vi "_033.vi"() -> ()   [LabVIEW 2024]
panel:
  out "Min":dbl
  out "Max":dbl
  in  "Array 4":dbl[](array[numeric])
  out "sum":dbl
  in  "Array 3":dbl[](array[numeric])
  out "x != 0?":bool
  out "x = 0?":bool
  in  "Numeric":dbl
  out "Array 2":dbl[](array[numeric])
  out "Array":dbl[](array[numeric])
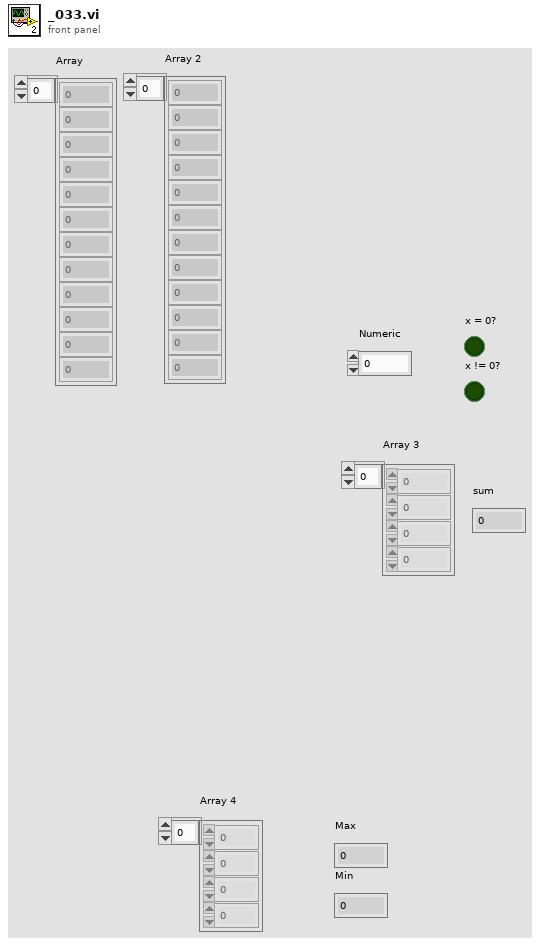
[diagram p1: front panel]
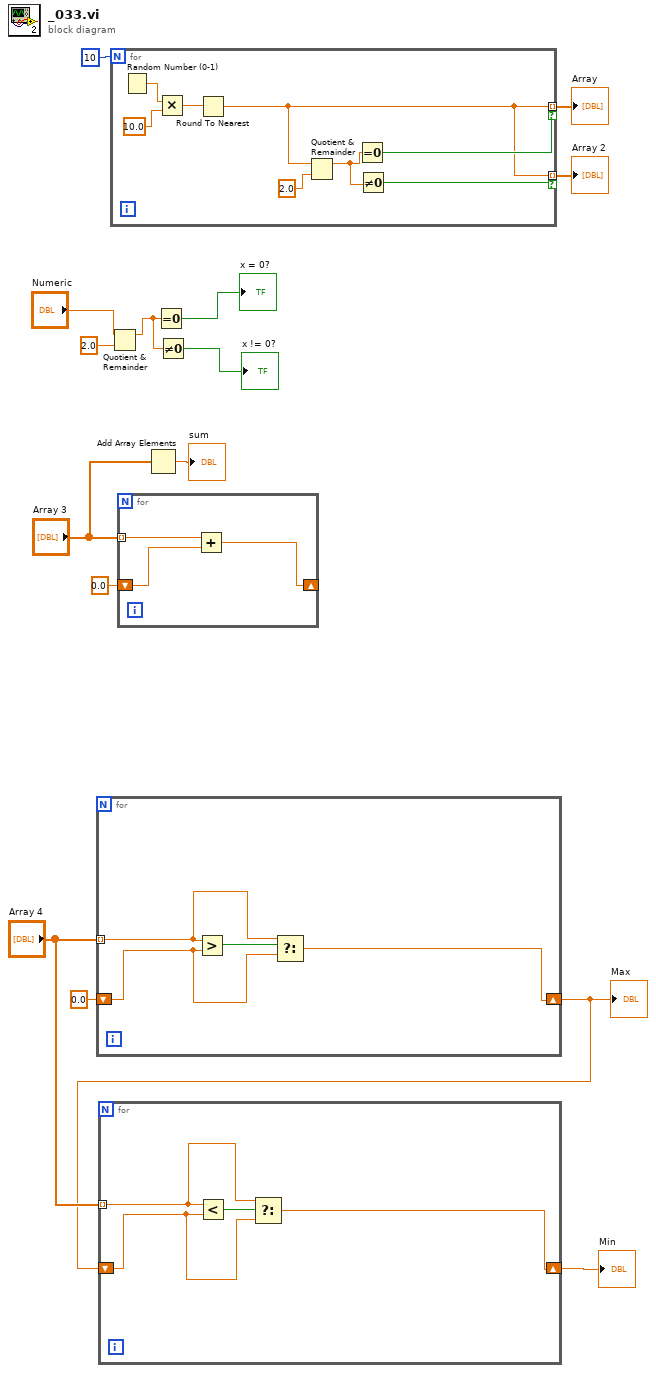
[diagram p0: block diagram]
diagram:
  n1 = for {
    tunnel: "Array 4" -> [w18] mode=indexing
    shift-right: [w17] -> w2
    shift-left: 0.0 ("Numeric") -> [w16]
    n2 = Greater?(x=w18, y=w16) -> (0:w19:bool)
    n3 = Select(t=w18, s=w19, f=w16) -> (s? t:f=w17:dbl)
  }
  "Max" <- w2
  n4 = for {
    tunnel: "Array 4" -> [w21] mode=indexing
    shift-right: [w22] -> w1
    shift-left: w2 -> [w20]
    n5 = Less?(x=w21, y=w20) -> (x < y?=w23:bool)
    n6 = Select(t=w21, s=w23, f=w20) -> (s? t:f=w22:dbl)
  }
  "Min" <- w1
  n7 = Quotient & Remainder(x="Numeric", y=2.0) -> (x-y*floor(x/y)=w10:dbl)  [unwired: 1 out]
  n8 = for {
    N: 10 -> [_]
    tunnel: [w25] -> w14 mode=indexing if=w28
    tunnel: [w25] -> w13 mode=indexing if=w27
    n9 = Random Number (0-1)() -> (number: 0 to 1=w31:dbl)
    n10 = Multiply(x=w31, y=10.0) -> (x*y=w29:dbl)
    n11 = Round To Nearest(number=w29) -> (nearest integer value=w25:dbl)
    n12 = Quotient & Remainder(x=w25, y=2.0) -> (x-y*floor(x/y)=w26:dbl)  [unwired: 1 out]
    n13 = Equal To 0?(x=w26) -> (x = 0?=w28:bool)
    n14 = Not Equal To 0?(x=w26) -> (x != 0?=w27:bool)
  }
  "Array" <- w14
  "Array 2" <- w13
  n15 = for {
    tunnel: "Array 3" -> [w34] mode=indexing
    shift-right: [w32] -> _
    shift-left: 0.0 -> [w33]
    n16 = Add(x=w34, y=w33) -> (x+y=w32:dbl)
  }
  n17 = Add Array Elements(numeric array="Array 3") -> (sum=→"sum":dbl)
  n18 = Equal To 0?(x=w10) -> (x = 0?=→"x = 0?":bool)
  n19 = Not Equal To 0?(x=w10) -> (x != 0?=→"x != 0?":bool)
